vi "Get I64.vi"(8 "error in (no error)":errorcluster, 10 "Offset":i32, 11 "JSON":string) -> (0 "error out":errorcluster, 1 "Number":i64)   [LabVIEW 2013, in "JSONtext.lvlib"]
uses:
  JSONtext.lvlib
  String Subset.vi
  Advance past Number.vi
  Parsing Error.vi
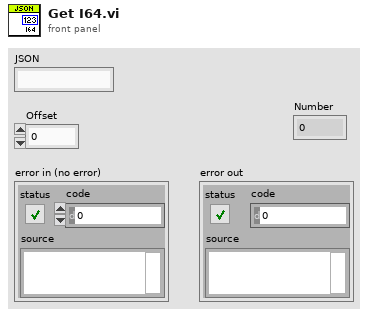
[diagram p1: front panel]
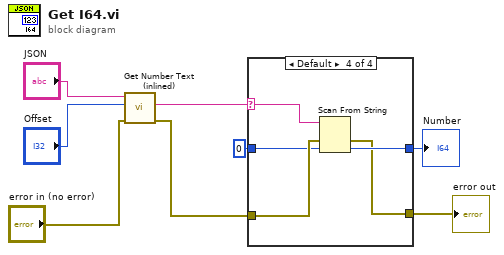
[diagram p0: block diagram]
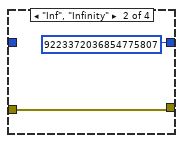
[diagram p3: hidden frame]
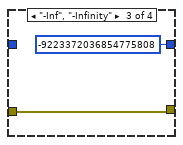
[diagram p4: hidden frame]
diagram:
  n1 = call "Get Number Text (inlined).vi"("error in (no error)"="error in (no error)", "Offset"="Offset", "JSON"="JSON") -> ("error out"=w4:errorcluster, "Number Text"=w2:string)  [unwired: 6 in, 1 out]
  n2 = case shown="Default" w2 {
    selector: w2 -> [_ _ _ w15]
    tunnel: [w9 i64 9223372036854775807 ("default value 1") i64 -9223372036854775808 ("default value 1") w19] -> w1
    tunnel: w4 -> [w10 w11 w13 w18]
    tunnel: [w10 w11 w13 w17] -> w3
    tunnel: i64 0 ("default value 1") -> [w9 _ _ w16]
    frame "NaN", "null" {
    }
    frame "Inf", "Infinity" {
    }
    frame "-Inf", "-Infinity" {
    }
    frame Default {
      n3 = Scan From String(input string=w15, error in=w18, default 1=w16) -> (error out=w17:errorcluster, output 1=w19:i64)  [unwired: 2 in, 2 out]
    }
  }
  "error out" <- w3
  "Number" <- w1
